vi "AudioStreamer.TrainTest.vi"(7 "trainer":bool, 11 "error in (no error)":errorcluster) -> (15 "error out":errorcluster)   [LabVIEW 2020]
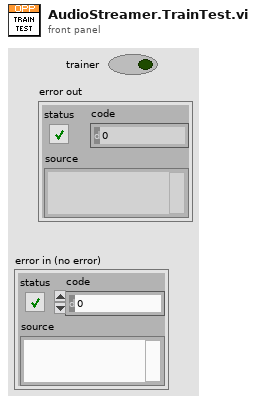
[diagram p1: front panel]
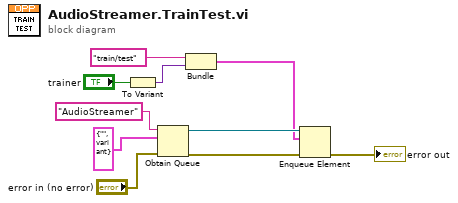
[diagram p0: block diagram]
diagram:
  n1 = To Variant(anything="trainer") -> (Variant=w1:variant)
  n2 = Obtain Queue(name (unnamed)="AudioStreamer", element data type=cluster{string, variant} {"", variant}, error in (no error)="error in (no error)") -> (queue out=w7:refnum<queue>, error out=w8:errorcluster)  [unwired: 2 in, 1 out]
  n3 = Bundle("train/test", "Variant"=w1) -> (w5:cluster{string, "Variant":variant})  [unwired: 1 in]
  n4 = Enqueue Element(queue=w7, element=w5, error in (no error)=w8) -> (error out=→"error out":errorcluster)  [unwired: 1 in, 2 out]
